vi "ControlFactory.vi"(8 "error in":errorcluster, 11 "Gen Refnum":refnum<vi>) -> (0 "error out":errorcluster, 3 "Control out":refnum<class "Control.lvclass">)   [LabVIEW 2014, in "Raspberry Pi Compatible Compiler for LabVIEW.lvlib" / "Control.lvclass"]
uses:
  Control.lvclass
  String/String.lvclass
  Boolean/Boolean.lvclass
  Tab/Tab.lvclass
  Numeric/Numeric.lvclass
  Cluster/Cluster.lvclass
  Path/Path.lvclass
  Array/Array.lvclass
  VisaResourceName/VisaResourceName.lvclass
  GraphChart/GraphChart.lvclass
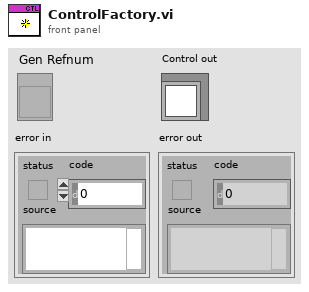
[diagram p1: front panel]
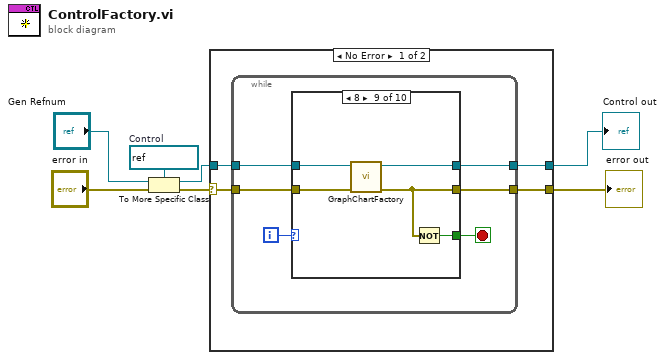
[diagram p0: block diagram]
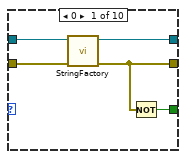
[diagram p2: hidden frame]
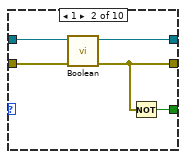
[diagram p3: hidden frame]
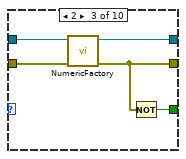
[diagram p4: hidden frame]
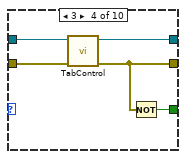
[diagram p5: hidden frame]
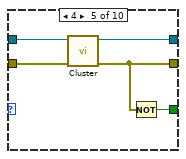
[diagram p6: hidden frame]
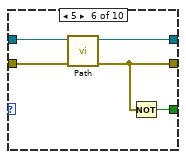
[diagram p7: hidden frame]
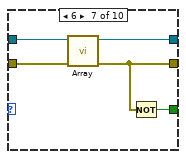
[diagram p8: hidden frame]
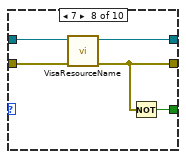
[diagram p9: hidden frame]
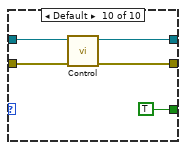
[diagram p10: hidden frame]
diagram:
  w6 = refnum<vi> refnum  # Control
  n1 = To More Specific Class(target class=w6, reference="Gen Refnum", error in="error in") -> (specific class reference=w3:refnum<vi>, error out=w4:errorcluster)
  n2 = case shown="No Error" w4 {
    selector: w4 -> [w11 w68]
    tunnel: [w9 _] -> w2
    tunnel: [w8 w68] -> w1
    tunnel: w3 -> [w10 _]
    frame No Error {
      n3 = while {
        tunnel: w11 -> [w16]
        tunnel: [w15] -> w8
        tunnel: [w14] -> w9
        tunnel: w10 -> [w12]
        i -> [w17]
        stop <- w13 stop-if-true
        n4 = case shown="8" w17 {
          tunnel: w16 -> [w22 w27 w32 w37 w42 w47 w52 w57 w62 w65]
          tunnel: [w19 w24 w29 w34 w39 w44 w49 w54 w59 w63] -> w15
          tunnel: [w21 w26 w31 w36 w41 w46 w51 w56 w61 w64] -> w14
          tunnel: [w20 w25 w30 w35 w40 w45 w50 w55 w60 TRUE] -> w13
          tunnel: w12 -> [w18 w23 w28 w33 w38 w43 w48 w53 w58 w66]
          frame 0 {
            n5 = call "StringFactory.vi"("error in"=w22, "reference"=w18) -> ("error out"=w19:errorcluster, "String out"=w21:refnum<class "String.lvclass">)  [unwired: 8 in]
            n6 = Not(x=w19) -> (.not. x?=w20:bool)
          }
          frame 1 {
            n7 = call "Boolean.vi"("error in"=w27, "GObj Refnum"=w23) -> ("error out"=w24:errorcluster, "Boolean out"=w26:refnum<class "Boolean.lvclass">)  [unwired: 8 in]
            n8 = Not(x=w24) -> (.not. x?=w25:bool)
          }
          frame 2 {
            n9 = call "NumericFactory.vi"("error in"=w32, "Gen Refnum"=w28) -> ("error out"=w29:errorcluster, "Numeric out"=w31:refnum<class "Numeric.lvclass">)  [unwired: 8 in]
            n10 = Not(x=w29) -> (.not. x?=w30:bool)
          }
          frame 3 {
            n11 = call "TabControl.vi"("error in"=w37, "Gen Refnum"=w33) -> ("error out"=w34:errorcluster, "Tab out"=w36:refnum<class "Tab.lvclass">)  [unwired: 8 in]
            n12 = Not(x=w34) -> (.not. x?=w35:bool)
          }
          frame 4 {
            n13 = call "Cluster.vi"("error in"=w42, "Gen Refnum"=w38) -> ("error out"=w39:errorcluster, "Cluster out"=w41:refnum<class "Cluster.lvclass">)  [unwired: 8 in]
            n14 = Not(x=w39) -> (.not. x?=w40:bool)
          }
          frame 5 {
            n15 = call "Path.vi"("error in"=w47, "Path in"=w43) -> ("error out"=w44:errorcluster, "Path out"=w46:refnum<class "Path.lvclass">)  [unwired: 8 in]
            n16 = Not(x=w44) -> (.not. x?=w45:bool)
          }
          frame 6 {
            n17 = call "Array.vi"("error in"=w52, "Gen Refnum"=w48) -> ("error out"=w49:errorcluster, "Array out"=w51:refnum<class "Array.lvclass">)  [unwired: 8 in]
            n18 = Not(x=w49) -> (.not. x?=w50:bool)
          }
          frame 7 {
            n19 = call "VisaResourceName.vi"("error in"=w57, "Refnum"=w53) -> ("error out"=w54:errorcluster, "VisaResourceName"=w56:refnum<class "VisaResourceName.lvclass">)  [unwired: 8 in]
            n20 = Not(x=w54) -> (.not. x?=w55:bool)
          }
          frame 8 {
            n21 = call "GraphChartFactory.vi"("error in"=w62, "Gen Refnum"=w58) -> ("error out"=w59:errorcluster, "GraphChart out"=w61:refnum<class "GraphChart.lvclass">)  [unwired: 8 in]
            n22 = Not(x=w59) -> (.not. x?=w60:bool)
          }
          frame Default {
            n23 = call "Control.vi"("error in"=w65, "GObj Refnum"=w66) -> ("error out"=w63:errorcluster, "Control out"=w64:refnum<class "Control.lvclass">)  [unwired: 8 in]
          }
        }
      }
    }
    frame Error {
    }
  }
  "error out" <- w1
  "Control out" <- w2
